vi "Actuator main.vi"() -> ()   [LabVIEW 2016]
uses:
  General/Controls/Queue modes.ctl
  General/Controls/staus modes.ctl
  General/Controls/Test settings.ctl
  General/Controls/References.ctl
  General/Controls/State control cluster.ctl
  General/Controls/States.ctl
  Actuator/Controls/Command cluster.ctl
  Actuator/Controls/Command list.ctl
  Actuator/Controls/Actuator fgv modes.ctl
  Webcam/Controls/Camera queue.ctl
  Webcam/Controls/Camera states.ctl
  DAQ/Controls/DAQ queue.ctl
  DAQ/Controls/Queue states.ctl
  <vilib>/Utility/cursorutil.llb/Set Cursor (Icon Pict).vi
  <vilib>/Platform/browser.llb/Open URL in Default Browser (string).vi
panel:
  out "Initialised":bool
  out "Trigger":bool
  in  "Load method":bool
  out "Logo 1":picture
  out "Logo 2":picture
  in  "Zero":bool
  in  "Load cell setup":bool
  in  "Abort move":bool
  in  "Initalise":bool
  in  "Snap image":bool
  in  "Test setup":bool
  in  "Camera setup":bool
  in  "Actuator setup":bool
  in  "Connect DAQ":bool
  in  "Test":bool
  in  "Connect Camera":bool
  in  "Connect Actuator":bool caption="IVIUM"
  in  "String":string=" \nLive data"
  out "LIVE DATA":dbl[](graph)
  out "LIVE DATA Force":dbl[](graph)
  in  "String 2":string=" \nActuator control"
  in  "Tab Control":enum32{"Blank", "Actuator interface"}(tab)
  in  "Limit position":dbl caption="mm" min=0.0 max=300.0 step=0.0001
  in  "Home":bool
  in  "Up":bool caption="Jog"
  in  "Down":bool
  in  "Speed":dbl=0.0001 caption="mm/s" min=0.0001 max=20.0 step=0.0001
  in  "Move absolute":bool
  in  "Target position":dbl caption="mm"
  in  "Home position":dbl caption="mm" min=0.0 max=300.0 step=0.0001
  out "Current position":dbl format="Current position - %8.4f mm"
  in  "Run method":bool
  in  "String 3":string=" \nTest data"
  out "TEST DATA":cluster{"Value":dbl, "data":dbl}(graph)
  in  "Status":string="©ReSolve Research Engineering Ltd. 2017"
  in  "Copright notice":string="Copright"
  # "Connections"
  # "Settings"
  # "Controls"
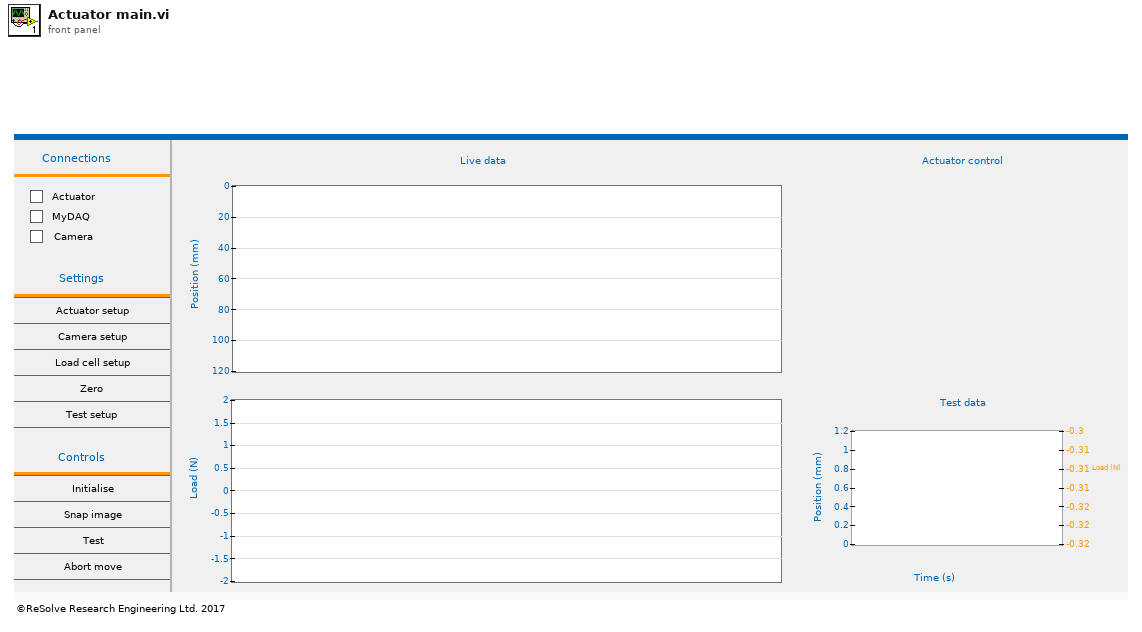
[diagram p1: front panel]
types:
  T1 = typedef "References.ctl" = cluster{"Tab Control":refnum<vi>, "Logo 1":refnum<vi>, "Logo 2":refnum<vi>, "Connect Actuator":refnum<vi>, "LIVE DATA":refnum<vi>, "Speed":refnum<vi>, "Home position":refnum<vi>, "Limit position":refnum<vi>, "Trigger":refnum<vi>, "Current position":refnum<vi>, "Connect Camera":refnum<vi>, "TEST DATA":refnum<vi>, "LIVE DATA Force":refnum<vi>, "Connect DAQ":refnum<vi>, "Initialised":refnum<vi>, "Test":refnum<vi>}
  T2 = typedef "Test settings.ctl" = cluster{"Speed (mm/s)":dbl, "Position limit":bool, "Position limit (mm)":dbl, "Load limit":bool, "Load limit (N)":dbl, "No. of repeats":u16, "Test identifier":string, "Time wait":bool, "Wait time (s)":dbl, "Trigger wait":bool, "Send trigger":bool, "Test notes":string, "Snap intervals":bool, "Time interval (s)":dbl}
  T3 = typedef "staus modes.ctl" = enum16{"Status", "Testing", "Webcam", "DAQ", "Actuator", "Initialise"}
  T4 = typedef "Queue modes.ctl" = enum16{"Initialise", "Destroy", "Get"}
  T5 = typedef "UEs.ctl" = cluster{"Read position":refnum<user-event>, "Check home":refnum<user-event>, "Record":refnum<user-event>, "Abort controller":refnum<user-event>, "Remote test":refnum<user-event>, "Test setup":refnum<user-event>, "Conditional wait":refnum<user-event>, "Abort move":refnum<user-event>, "Wait done":refnum<user-event>, "Send trigger":refnum<user-event>, "Initalising":refnum<user-event>, "Initalisation complete":refnum<user-event>}
  T6 = typedef "State control cluster.ctl" = cluster{"State":T7, "Data":variant}
  T7 = typedef "States.ctl" = enum16{"Initialise", "Actuator connection", "Get info", "Send command", "Load method", "Run method", "Save test", "Setup", "Shutdown"}
  T8 = typedef "Actuator fgv modes.ctl" = enum16{"Initalise", "COM", "Limit", "Speed", "Home", "Get"}
  T9 = typedef "Command cluster.ctl" = cluster{"Command":T10, "data":variant}
  T10 = typedef "Command list.ctl" = enum16{"", "£nabort", "getaxisno", "£getserialno", "£nidentify", "&&£setnlimit", "&£nm", "&£snv", "&£speed", "£np", "£ncal"}
  T11 = typedef "Camera queue.ctl" = cluster{"State":T12, "Data":variant}
  T12 = typedef "Camera states.ctl" = enum16{"Initialise", "Setup", "Connect", "Snap", "Close", "Shutdown"}
  T13 = typedef "DAQ queue.ctl" = cluster{"Sate":T14, "Data":variant}
  T14 = typedef "Queue states.ctl" = enum16{"Shutdown", "Save data", "Record", "Read", "Setup", "Zero", "Connect", "Initialise"}
  T15 = typedef "Default settings.ctl" = cluster{"COM port":refnum<visa-resource-name>, "Home pos":dbl, "Speed":dbl, "Limit stop":dbl}
  T16 = typedef "LVCursorListTypeDef.ctl" = cluster{"Name":string, "Color":u32, "Style":u8, "Point Style":u8, "Name Visible":bool, "Allow Drag":bool, "Cursor Mode":u32, "Plot":i32, "Index":i32, "Position":cluster{"X":dbl, "Y":dbl}, "X Scale":u32, "Y Scale":u32, "Watch Plots":i32[], "Watch All Plots":bool, "Plot Area":i32, "Label Offset":cluster{"X":dbl, "Y":dbl}}[]
  T17 = cluster{"Name":string, "Color":u32, "Style":u8, "Point Style":u8, "Name Visible":bool, "Allow Drag":bool, "Cursor Mode":u32, "Plot":i32, "Index":i32, "Position":cluster{"X":dbl, "Y":dbl}, "X Scale":u32, "Y Scale":u32, "Watch Plots":i32[], "Watch All Plots":bool, "Plot Area":i32, "Label Offset":cluster{"X":dbl, "Y":dbl}}
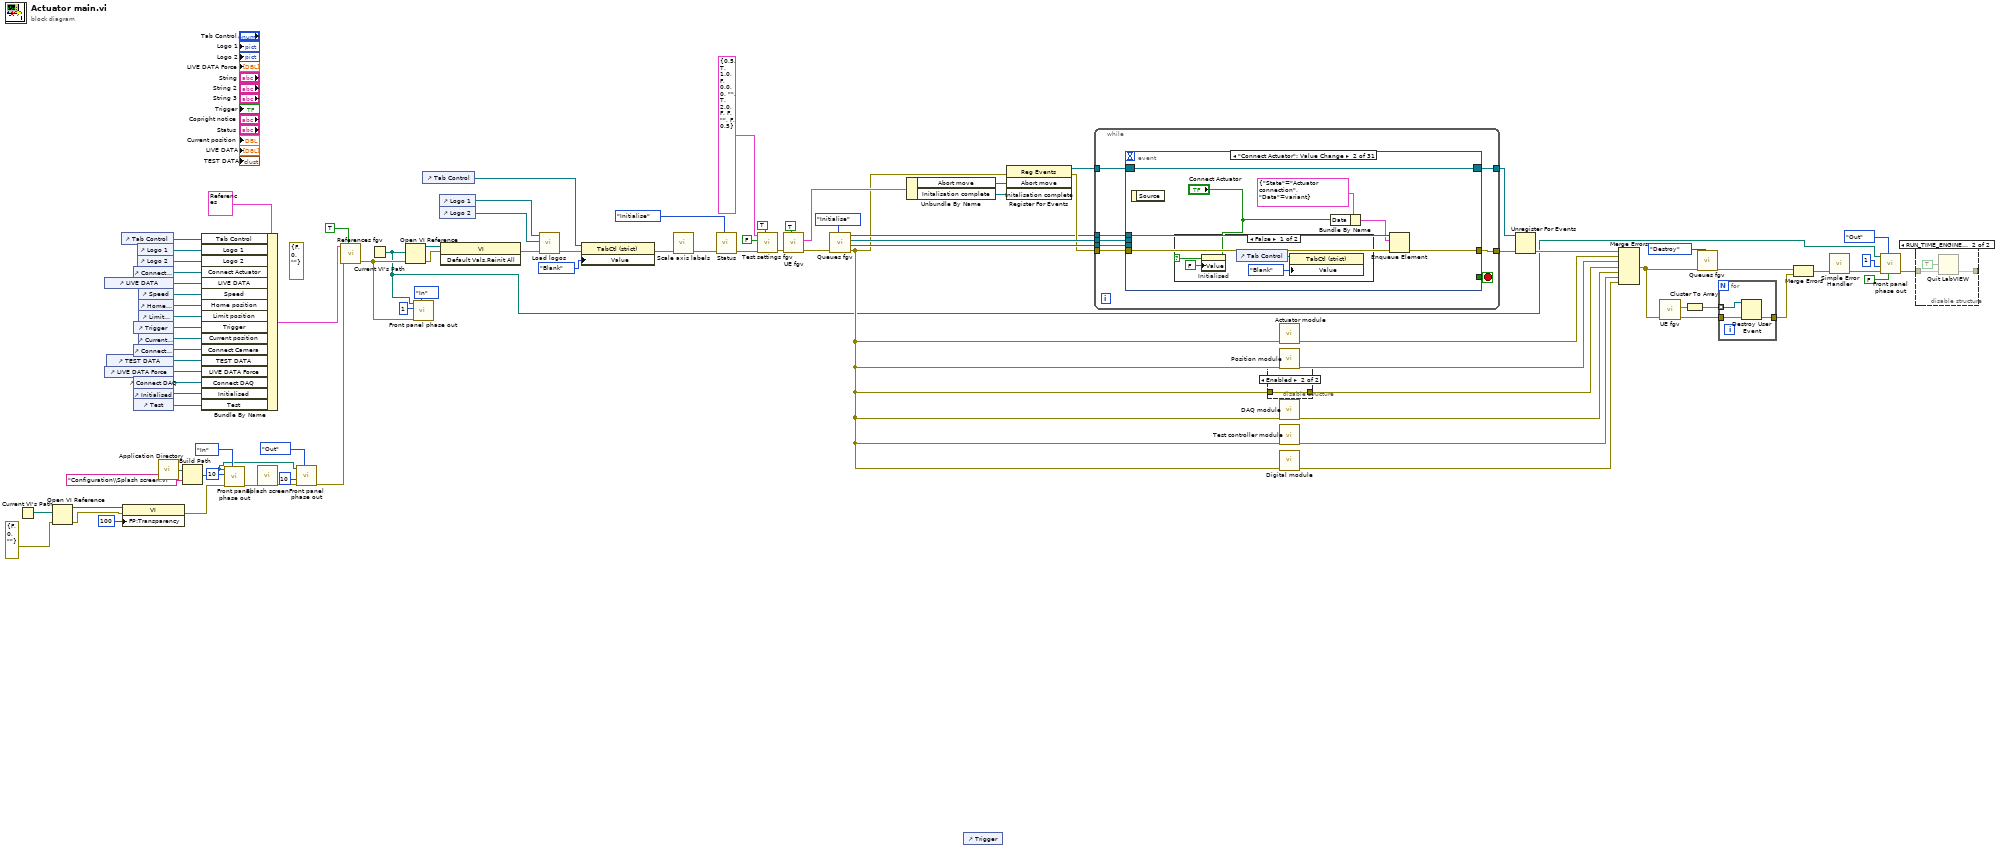
[diagram p0: block diagram]
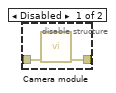
[diagram p2: hidden frame]
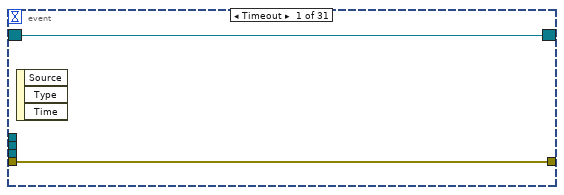
[diagram p4: hidden frame]
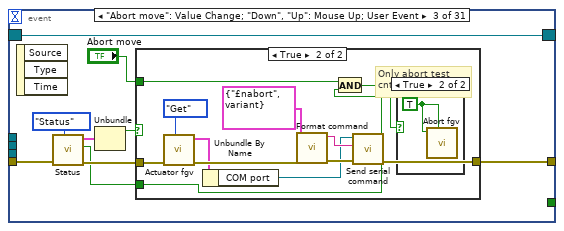
[diagram p6: hidden frame]
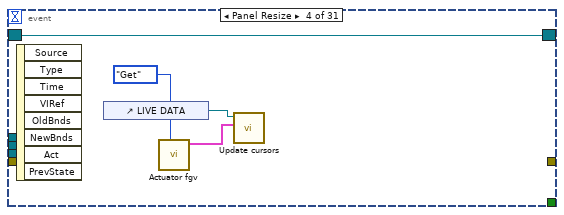
[diagram p9: hidden frame]
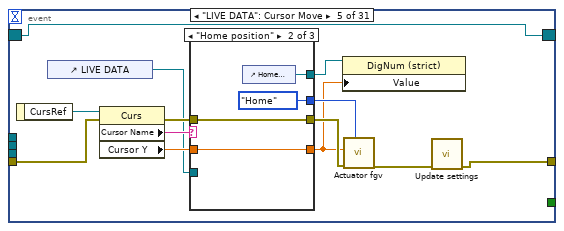
[diagram p10: hidden frame]
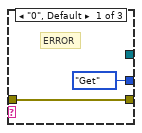
[diagram p11: hidden frame]
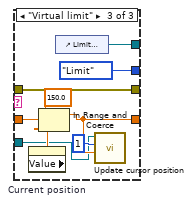
[diagram p12: hidden frame]
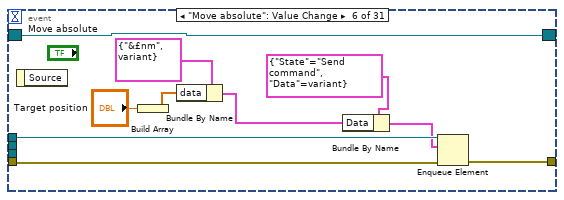
[diagram p13: hidden frame]
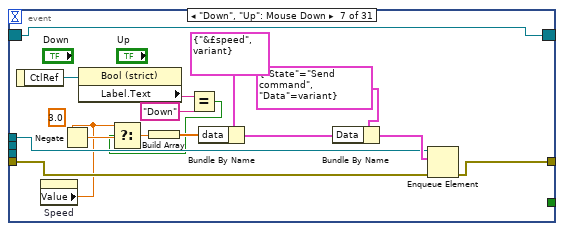
[diagram p14: hidden frame]
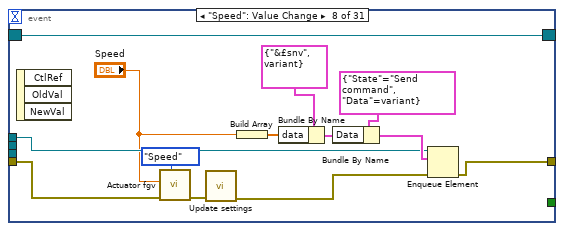
[diagram p15: hidden frame]
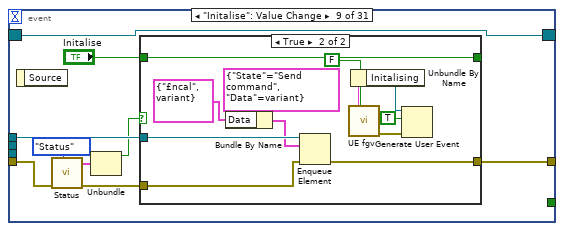
[diagram p16: hidden frame]
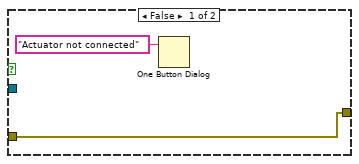
[diagram p17: hidden frame]
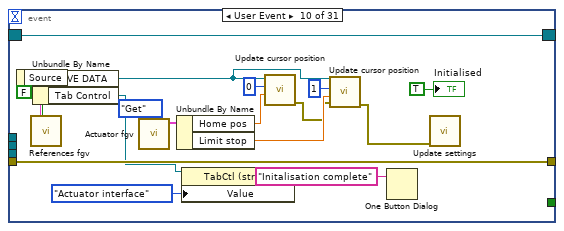
[diagram p18: hidden frame]
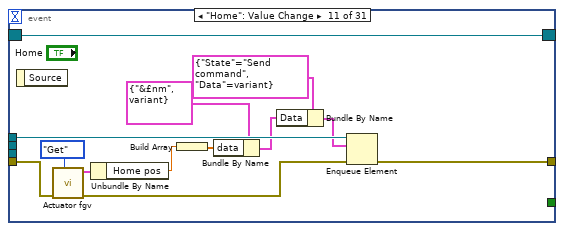
[diagram p19: hidden frame]
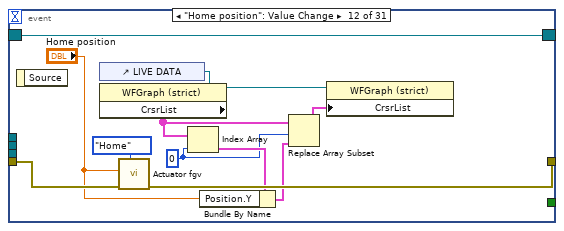
[diagram p20: hidden frame]
diagram:
  (unwired) errorcluster {"status"=FALSE, "code"=0, "source"=""} ("error in (no error)")
  n1 = Current VI's Path() -> (path=w16:path)
  n2 = Open VI Reference(vi path=w16, error in (no error)=errorcluster {"status"=FALSE, "code"=0, "source"=""}) -> (vi reference=w13:refnum<vi>, error out=w5:errorcluster)  [unwired: 4 in]
  n3 = control-ref of="LIVE DATA"() -> (w51:refnum<vi>)
  n4 = control-ref of="LIVE DATA Force"() -> (w41:refnum<vi>)
  n5 = control-ref of="TEST DATA"() -> (w42:refnum<vi>)
  n6 = control-ref of="Tab Control"() -> (w55:refnum<vi>)
  n7 = property class="VI"(reference=w13, error in=w5, "FP:Transparency"=u8 100 ("Front Panel Window:Transparency")) -> (error out=w12:errorcluster)  [unwired: 1 out]
  n8 = control-ref of="Connect Actuator"() -> (w52:refnum<vi>)
  n9 = control-ref of="Trigger"() -> (w45:refnum<vi>)
  n10 = control-ref of="Connect Camera"() -> (w43:refnum<vi>)
  n11 = control-ref of="Connect DAQ"() -> (w40:refnum<vi>)
  n12 = control-ref of="Initialised"() -> (w39:refnum<vi>)
  n13 = control-ref of="Test"() -> (w38:refnum<vi>)
  n14 = control-ref of="Logo 1"() -> (w54:refnum<vi>)
  n15 = control-ref of="Logo 2"() -> (w53:refnum<vi>)
  n16 = control-ref of="Speed"() -> (w50:refnum<vi>)
  n17 = control-ref of="Home position"() -> (w49:refnum<vi>)
  n18 = control-ref of="Limit position"() -> (w48:refnum<vi>)
  n19 = control-ref of="Current position"() -> (w44:refnum<vi>)
  n20 = call <vilib>:"Application Directory.vi"() -> ("Application Directory"=w27:path)
  n21 = Build Path(base path=w27, name or relative path="Configuration\\Splash screen.vi") -> (appended path=w22:path)
  n22 = Bundle By Name(cluster=T1 {"Tab Control"=refnum, "Logo 1"=refnum, "Logo 2"=refnum, "Connect Actuator"=refnum, "LIVE DATA"=refnum, "Speed"=refnum, "Home position"=refnum, "Limit position"=refnum, "Trigger"=refnum, "Current position"=refnum, "Connect Camera"=refnum, "TEST DATA"=refnum, "LIVE DATA Force"=refnum, "Connect DAQ"=refnum, "Initialised"=refnum, "Test"=refnum}, "Tab Control"=w55, "Logo 1"=w54, "Logo 2"=w53, "Connect Actuator"=w52, "LIVE DATA"=w51, "Speed"=w50, "Home position"=w49, "Limit position"=w48, "Trigger"=w45, "Current position"=w44, "Connect Camera"=w43, "TEST DATA"=w42, "LIVE DATA Force"=w41, "Connect DAQ"=w40, "Initialised"=w39, "Test"=w38) -> (w47:T1)
  n23 = call "Front panel phase out.vi"("Mode"=enum16{"In", "Out"}."In", "error in (no error)"=w12, "millisecond multiple In"=u32 10, "path"=w22) -> ("error out"=w24:errorcluster)  [unwired: 7 in]
  n24 = call "Splash screen.vi"("error in (no error)"=w24) -> ("error out"=w23:errorcluster)  [unwired: 10 in]
  n25 = call "Front panel phase out.vi"("Mode"=enum16{"In", "Out"}."Out", "error in (no error)"=w23, "millisecond multiple out"=u32 10, "path"=w22) -> ("error out"=w20:errorcluster)  [unwired: 7 in]
  n26 = call "References fgv.vi"("Set?"=TRUE, "error in (no error)"=w20, 11:w47) -> ("error out"=w19:errorcluster)  [unwired: 7 in, 1 out]
  n27 = Current VI's Path() -> (path=w9:path)
  n28 = Open VI Reference(vi path=w9, error in (no error)=w19) -> (vi reference=w18:refnum<vi>, error out=w89:errorcluster)  [unwired: 4 in]
  n29 = call "Front panel phase out.vi"("Mode"=enum16{"In", "Out"}."In", "error in (no error)"=w19, "millisecond multiple In"=u32 1, "path"=w9) -> ()  [unwired: 7 in, 1 out]
  n30 = control-ref of="Tab Control"() -> (w83:refnum<vi>)
  n31 = control-ref of="Logo 1"() -> (w65:refnum<vi>)
  n32 = control-ref of="Logo 2"() -> (w64:refnum<vi>)
  n33 = invoke class="VI" method="Default Vals.Reinit All"(reference=w18, error in=w89) -> (error out=w33:errorcluster)  [unwired: 1 in, 2 out]
  n34 = call "Load logos.vi"("error in (no error)"=w33, "Logo 2"=w64, "Logo 1"=w65) -> ("error out"=w63:errorcluster)  [unwired: 6 in, 2 out]
  n35 = property class="TabCtl (strict)"(reference=w83, error in=w63, "Value"=enum32{"Blank", "Actuator interface"}."Blank") -> (error out=w32:errorcluster)  [unwired: 1 out]
  n36 = call "Scale axis labels.vi"("error in (no error)"=w32) -> ("error out"=w31:errorcluster)  [unwired: 10 in]
  n37 = call "Status.vi"("Mode"=staus_modes."Initialise", "error in (no error)"=w31) -> ("error out"=w70:errorcluster)  [unwired: 7 in, 2 out]
  n38 = call "Test settings fgv.vi"("Set?"=TRUE, "error in (no error)"=w70, "Settings selected?"=FALSE, "Test settings"=T2 {"Speed (mm/s)"=0.5, "Position limit"=TRUE, "Position limit (mm)"=1.0, "Load limit"=FALSE, "Load limit (N)"=0.0, "No. of repeats"=0, "Test identifier"="", "Time wait"=TRUE, "Wait time (s)"=2.0, "Trigger wait"=FALSE, "Send trigger"=FALSE, "Test notes"="", "Snap intervals"=FALSE, "Time interval (s)"=0.5}) -> ("error out"=w37:errorcluster)  [unwired: 5 in, 2 out]
  n39 = call "UE fgv.vi"("Set?"=TRUE, "error in (no error)"=w37) -> ("error out"=w36:errorcluster, "UEs"=w35:T5)  [unwired: 7 in, 1 out]
  n40 = call "Queues fgv.vi"("Modes"=Queue_modes."Initialise", "error in (no error)"=w36) -> ("error in (no error) 2"=w34:errorcluster, "DAQ"=w81:refnum<queue>, "Camera"=w87:refnum<queue>, "Ivium"=w61:refnum<queue>)  [unwired: 6 in]
  n41 = Unbundle By Name(w35) -> ("Abort move"=w72:refnum<user-event>, "Initalisation complete"=w1:refnum<user-event>)
  n42 = control-ref of="Trigger"() -> ()  [unwired: 1 out]
  n43 = register-events(error in=w34, w72, w1) -> (reference out=w71:refnum<event-registration>, error out=w66:errorcluster)  [unwired: 1 in]
  n44 = while {
    tunnel: w66 -> [w96]
    tunnel: [w95] -> w59
    tunnel: w61 -> [w94]
    tunnel: w87 -> [w93]
    tunnel: w81 -> [w92]
    tunnel: w71 -> [w91]
    tunnel: [w90] -> w57
    stop <- w97 stop-if-true
    n45 = event shown="[1] \"Connect Actuator\": Value Change" {
      selector: w91 -> [w98 w101 w111 w133 w137 w165 w175 w191 w204 w243 w244 w257 w269 w282 w287 w292 w299 w306 w311 w316 w321 w326 w331 w339 w347 w351 w355 w359 w363 w368 w373]
      dyn-events: [w98 w101 w111 w133 w137 w165 w175 w191 w204 w243 w244 w257 w269 w282 w287 w292 w299 w306 w311 w316 w321 w326 w331 w339 w347 w351 w355 w359 w363 w368 w373] -> w90
      timeout: _ -> [_ _ _ _ _ _ _ _ _ _ _ _ _ _ _ _ _ _ _ _ _ _ _ _ _ _ _ _ _ _ _]
      tunnel: [_ _ _ _ _ _ _ _ _ _ _ _ _ _ _ _ _ _ _ _ _ _ _ _ _ _ _ _ _ _ TRUE] -> w97
      tunnel: w96 -> [w99 w106 w115 _ w143 w166 w184 w196 w210 w242 w249 w268 w281 w283 w291 w298 w305 w310 w315 w320 w325 w330 w335 w343 w349 w353 w356 w362 w366 w371 w377]
      tunnel: [w99 w104 w118 _ w141 w171 w185 w198 w212 w242 w256 w266 w277 w285 w289 w297 w304 w309 w314 w319 w324 w327 w338 w346 w348 w352 w357 w361 w365 w370 w380] -> w95
      tunnel: w94 -> [_ w105 _ _ _ w170 w183 w197 w211 _ w255 _ _ w286 w290 _ _ _ _ _ _ w329 _ _ _ _ _ _ _ _ w390]
      tunnel: w93 -> [_ _ _ _ _ _ _ _ _ _ _ _ _ _ _ w295 _ w308 _ _ w323 _ _ _ _ _ _ _ _ _ w388]
      tunnel: w92 -> [_ _ _ _ _ _ _ _ _ _ _ _ _ _ _ _ w301 _ w313 w318 _ _ _ _ _ _ _ _ _ _ w386]
      event Timeout {
        n46 = event-data() -> ()  [unwired: 1 in, 3 out]
      }
      event "Connect Actuator": Value Change {
        n47 = event-data() -> ()  [unwired: 1 in, 1 out]
        n48 = case shown="False" "Connect Actuator" {
          frame False {
            n49 = property on="Initialised" class="Bool (strict)"("Value"=FALSE ("Initialised")) -> ()  [unwired: 2 in, 2 out]
            n50 = control-ref of="Tab Control"() -> (w109:refnum<vi>)
            n51 = property class="TabCtl (strict)"(reference=w109, "Value"=enum32{"Blank", "Actuator interface"}."Blank") -> ()  [unwired: 1 in, 2 out]
          }
          frame True {
          }
        }
        n52 = Bundle By Name(cluster=T6 {"State"=enum."Actuator connection", "Data"=variant} ("State control"), "Data"="Connect Actuator") -> (w102:T6)
        n53 = Enqueue Element(queue=w105, element=w102, error in (no error)=w106) -> (error out=w104:errorcluster)  [unwired: 1 in, 2 out]
      }
      event "Abort move": Value Change; "Down", "Up": Mouse Up; User Event {
        n54 = event-data() -> ()  [unwired: 1 in, 3 out]
        n55 = call "Status.vi"("Mode"=staus_modes."Status", "error in (no error)"=w115) -> ("error out"=w114:errorcluster, "Testing"=w112:bool, "Connections"=w116:cluster{"Data":bool, "Data":bool, "Data":bool})  [unwired: 7 in]
        n56 = Unbundle(w116) -> ("Data"=w113:bool)  [unwired: 2 out]
        n57 = case shown="True" w113 {
          tunnel: [w119 w129] -> w118
          tunnel: w114 -> [w119 w128]
          tunnel: w112 -> [_ w121]
          tunnel: "Abort move" -> [_ w122]
          frame False {
          }
          frame True {
            # "Only abort test \ncntrl from button"
            n58 = call "Actuator fgv.vi"("Enum"=Actuator_fgv_modes."Get", "error in (no error)"=w128) -> ("error out"=w127:errorcluster, "Cluster out"=w125:T15)  [unwired: 8 in]
            n59 = Unbundle By Name(w125) -> ("COM port"=w123:refnum<visa-resource-name>)
            n60 = call "Format command.vi"("error in (no error)"=w127, "Cluster"=T9 {"Command"=enum."£nabort", "data"=variant}) -> ("error out"=w131:errorcluster, "String"=w130:string)  [unwired: 8 in]
            n61 = And(x=w122, y=w121) -> (x .and. y?=w120:bool)
            n62 = call "Send serial command.vi"("error IO"=w131, "Send string"=w130, "VISA resource name out"=w123) -> ("error out"=w129:errorcluster)  [unwired: 6 in, 2 out]
            n63 = case shown="True" w120 {
              frame False {
              }
              frame True {
                w132 = TRUE ("Set?")
                n64 = call "Abort fgv.vi"("Set?"=w132, "Value"=w132) -> ()  [unwired: 9 in, 1 out]
              }
            }
          }
        }
      }
      event Panel Resize {
        n65 = event-data() -> ()  [unwired: 1 in, 8 out]
        n66 = control-ref of="LIVE DATA"() -> (w134:refnum<vi>)
        n67 = call "Actuator fgv.vi"("Enum"=Actuator_fgv_modes."Get") -> ("Cluster out"=w135:T15)  [unwired: 9 in, 1 out]
        n68 = call "Update cursors.vi"("Cluster in"=w135, "LIVE DATA 3"=w134) -> ()  [unwired: 9 in, 1 out]
      }
      event "LIVE DATA": Cursor Move {
        n69 = event-data() -> ("CursRef"=w149:refnum<vi>)  [unwired: 1 in]
        n70 = control-ref of="LIVE DATA"() -> (w138:refnum<vi>)
        n71 = property class="Curs"(reference=w149, error in=w143) -> (error out=w145:errorcluster, "Cursor Name"=w148:string, "Cursor Y"=w147:dbl)  [unwired: 1 out]
        n72 = case shown="\"Home position\"" w148 {
          tunnel: w147 -> [_ w155 w161]
          tunnel: [_ w155 w158] -> w139
          tunnel: [Actuator_fgv_modes."Get" ("Enum") Actuator_fgv_modes."Home" ("Enum") Actuator_fgv_modes."Limit" ("Enum")] -> w146
          tunnel: w145 -> [w150 w153 w163]
          tunnel: [w150 w153 w163] -> w144
          tunnel: [_ w152 w162] -> w140
          tunnel: w138 -> [_ _ w156]
          frame "0", Default {
            # "ERROR"
          }
          frame "Home position" {
            n73 = control-ref of="Home position"() -> (w152:refnum<vi>)
          }
          frame "Virtual limit" {
            n74 = property on="Current position" class="DigNum (strict)"() -> ("Value"=w160:dbl)  [unwired: 2 in, 2 out]
            n75 = In Range and Coerce(upper limit=150.0, x=w161, lower limit=w160) -> (coerced(x)=w158:dbl)  [unwired: 1 out]
            n76 = control-ref of="Limit position"() -> (w162:refnum<vi>)
            n77 = call "Update cursor position.vi"("Position Y"=w158, "index"=1, "LIVE DATA 3"=w156) -> ()  [unwired: 8 in, 1 out]
          }
        }
        n78 = property class="DigNum (strict)"(reference=w140, "Value"=w139) -> ()  [unwired: 1 in, 2 out]
        n79 = call "Actuator fgv.vi"("Enum"=w146, "error in (no error)"=w144, "Data"=w139) -> ("error out"=w142:errorcluster)  [unwired: 7 in, 1 out]
        n80 = call "Update settings.vi"("error in (no error)"=w142) -> ("error out"=w141:errorcluster)  [unwired: 10 in]
      }
      event "Move absolute": Value Change {
        n81 = event-data() -> ()  [unwired: 1 in, 1 out]
        n82 = Build Array("Target position") -> (w172:dbl[])
        n83 = Bundle By Name(cluster=T9 {"Command"=enum."&£nm", "data"=variant} ("Cluster"), "data"=w172) -> (w168:T9)
        n84 = Bundle By Name(cluster=T6 {"State"=enum."Send command", "Data"=variant} ("element"), "Data"=w168) -> (w167:T6)
        n85 = Enqueue Element(queue=w170, element=w167, error in (no error)=w166) -> (error out=w171:errorcluster)  [unwired: 1 in, 2 out]
      }
      event "Down", "Up": Mouse Down {
        (unwired) 3.0
        n86 = event-data() -> ("CtlRef"=w180:refnum<vi>)  [unwired: 1 in]
        n87 = property on="Speed" class="DigNum (strict)"() -> ("Value"=w176:dbl)  [unwired: 2 in, 2 out]
        n88 = Negate(x=w176) -> (-x=w182:dbl)
        n89 = property class="Bool (strict)"(reference=w180) -> ("Label.Text"=w179:string)  [unwired: 1 in, 2 out]
        n90 = Equal?(x=w179, y="Down") -> (x = y?=w177:bool)
        n91 = Select(t=w176, s=w177, f=w182) -> (s? t:f=w181:dbl)
        n92 = Build Array(w181) -> (w190:dbl[])
        n93 = Bundle By Name(cluster=T9 {"Command"=enum."&£speed", "data"=variant} ("Cluster"), "data"=w190) -> (w186:T9)
        n94 = Bundle By Name(cluster=T6 {"State"=enum."Send command", "Data"=variant} ("element"), "Data"=w186) -> (w187:T6)
        n95 = Enqueue Element(queue=w183, element=w187, error in (no error)=w184) -> (error out=w185:errorcluster)  [unwired: 1 in, 2 out]
      }
      event "Speed": Value Change {
        n96 = event-data() -> ()  [unwired: 1 in, 3 out]
        n97 = call "Actuator fgv.vi"("Enum"=Actuator_fgv_modes."Speed", "error in (no error)"=w196, "Data"="Speed") -> ("error out"=w195:errorcluster)  [unwired: 7 in, 1 out]
        n98 = call "Update settings.vi"("error in (no error)"=w195) -> ("error out"=w194:errorcluster)  [unwired: 10 in]
        n99 = Build Array("Speed") -> (w203:dbl[])
        n100 = Bundle By Name(cluster=T9 {"Command"=enum."&£snv", "data"=variant} ("Cluster"), "data"=w203) -> (w199:T9)
        n101 = Bundle By Name(cluster=T6 {"State"=enum."Send command", "Data"=variant} ("element"), "Data"=w199) -> (w200:T6)
        n102 = Enqueue Element(queue=w197, element=w200, error in (no error)=w194) -> (error out=w198:errorcluster)  [unwired: 1 in, 2 out]
      }
      event "Initalise": Value Change {
        n103 = event-data() -> ()  [unwired: 1 in, 1 out]
        n104 = call "Status.vi"("Mode"=staus_modes."Status", "error in (no error)"=w210) -> ("error out"=w209:errorcluster, "Connections"=w208:cluster{"Data":bool, "Data":bool, "Data":bool})  [unwired: 7 in, 1 out]
        n105 = Unbundle(w208) -> ("Data"=w206:bool)  [unwired: 2 out]
        n106 = case shown="True" w206 {
          tunnel: [w213 w215] -> w212
          tunnel: w211 -> [_ w226]
          tunnel: w209 -> [w213 w222]
          tunnel: "Initalise" -> [_ w221]
          tunnel: [_ w221] -> _
          frame False {
            n107 = One Button Dialog(message="Actuator not connected") -> ()  [unwired: 1 in, 1 out]
          }
          frame True {
            n108 = Bundle By Name(cluster=T6 {"State"=enum."Send command", "Data"=variant} ("element"), "Data"=T9 {"Command"=enum."£ncal", "data"=variant} ("Cluster")) -> (w223:T6)
            n109 = Enqueue Element(queue=w226, element=w223, error in (no error)=w222) -> (error out=w215:errorcluster)  [unwired: 1 in, 2 out]
            n110 = call "UE fgv.vi"("Set?"=FALSE) -> ("error out"=w218:errorcluster, "UEs"=w219:T5)  [unwired: 8 in, 1 out]
            n111 = Unbundle By Name(w219) -> ("Initalising"=w217:refnum<user-event>)
            n112 = Generate User Event(user event=w217, event data cluster=TRUE ("event data"), error in=w218) -> ()  [unwired: 1 in, 2 out]
          }
        }
      }
      event User Event {
        n113 = event-data() -> ()  [unwired: 1 in, 1 out]
        n114 = call "References fgv.vi"("Set?"=FALSE) -> ("Cluster"=w239:T1)  [unwired: 9 in, 1 out]
        n115 = Unbundle By Name(w239) -> ("LIVE DATA"=w233:refnum<vi>, "Tab Control"=w238:refnum<vi>)
        n116 = call "Actuator fgv.vi"("Enum"=Actuator_fgv_modes."Get") -> ("Cluster out"=w235:T15)  [unwired: 9 in, 1 out]
        n117 = Unbundle By Name(w235) -> ("Home pos"=w234:dbl, "Limit stop"=w231:dbl)
        n118 = property class="TabCtl (strict)"(reference=w238, "Value"=enum32{"Blank", "Actuator interface"}."Actuator interface") -> ()  [unwired: 1 in, 2 out]
        n119 = call "Update cursor position.vi"("Position Y"=w234, "index"=0, "LIVE DATA 3"=w233) -> ("error out"=w229:errorcluster)  [unwired: 8 in]
        n120 = call "Update cursor position.vi"("error in (no error)"=w229, "Position Y"=w231, "index"=1, "LIVE DATA 3"=w233) -> ("error out"=w230:errorcluster)  [unwired: 7 in]
        n121 = One Button Dialog(message="Initalisation complete") -> ()  [unwired: 1 in, 1 out]
        n122 = call "Update settings.vi"("error in (no error)"=w230) -> ()  [unwired: 10 in, 1 out]
        "Initialised" <- TRUE ("Initialised")
      }
      event "Home": Value Change {
        n123 = event-data() -> ()  [unwired: 1 in, 1 out]
        n124 = call "Actuator fgv.vi"("Enum"=Actuator_fgv_modes."Get", "error in (no error)"=w249) -> ("error out"=w248:errorcluster, "Cluster out"=w246:T15)  [unwired: 8 in]
        n125 = Unbundle By Name(w246) -> ("Home pos"=w245:dbl)
        n126 = Build Array(w245) -> (w250:dbl[])
        n127 = Bundle By Name(cluster=T9 {"Command"=enum."&£nm", "data"=variant} ("Cluster"), "data"=w250) -> (w251:T9)
        n128 = Bundle By Name(cluster=T6 {"State"=enum."Send command", "Data"=variant} ("element"), "Data"=w251) -> (w253:T6)
        n129 = Enqueue Element(queue=w255, element=w253, error in (no error)=w248) -> (error out=w256:errorcluster)  [unwired: 1 in, 2 out]
      }
      event "Home position": Value Change {
        w262 = 0 ("index")
        n130 = event-data() -> ()  [unwired: 1 in, 1 out]
        n131 = control-ref of="LIVE DATA"() -> (w265:refnum<vi>)
        n132 = property class="WFGraph (strict)"(reference=w265) -> (reference out=w260:refnum<vi>, "CrsrList"=w263:T16)  [unwired: 1 in, 1 out]
        n133 = call "Actuator fgv.vi"("Enum"=Actuator_fgv_modes."Home", "error in (no error)"=w268, "Data"="Home position") -> ("error out"=w266:errorcluster)  [unwired: 7 in, 1 out]
        n134 = Index Array(array=w263, index=w262) -> (element=w264:T17)
        n135 = Bundle By Name(cluster=w264, "Position.Y"="Home position") -> (w261:T17)
        n136 = Replace Array Subset(array=w263, new element=w261, index=w262) -> (w259:T16)
        n137 = property class="WFGraph (strict)"(reference=w260, "CrsrList"=w259) -> ()  [unwired: 1 in, 2 out]
      }
      event "Limit position": Value Change {
        n138 = event-data() -> ()  [unwired: 1 in, 1 out]
        n139 = property on="Current position" class="DigNum (strict)"() -> ("Value"=w275:dbl)  [unwired: 2 in, 2 out]
        n140 = In Range and Coerce(upper limit=150.0, x="Limit position", lower limit=w275) -> (coerced(x)=w272:dbl)  [unwired: 1 out]
        n141 = control-ref of="LIVE DATA"() -> (w279:refnum<vi>)
        n142 = call "Actuator fgv.vi"("Enum"=Actuator_fgv_modes."Limit", "error in (no error)"=w281, "Data"=w272) -> ("error out"=w271:errorcluster)  [unwired: 7 in, 1 out]
        n143 = call "Update cursor position.vi"("error in (no error)"=w271, "Position Y"=w272, "index"=1, "LIVE DATA 3"=w279) -> ("error out"=w270:errorcluster)  [unwired: 7 in]
        n144 = property on="Limit position" class="DigNum (strict)"(error in=w270, "Value"=w272) -> (error out=w273:errorcluster)  [unwired: 1 in, 1 out]
        n145 = call "Update settings.vi"("error in (no error)"=w273) -> ("error out"=w277:errorcluster)  [unwired: 10 in]
      }
      event "Load method": Value Change {
        n146 = event-data() -> ()  [unwired: 1 in, 1 out]
        n147 = Enqueue Element(queue=w286, element=T6 {"State"=enum."Load method", "Data"=variant} ("State control"), error in (no error)=w283) -> (error out=w285:errorcluster)  [unwired: 1 in, 2 out]
      }
      event "Run method": Value Change {
        n148 = event-data() -> ()  [unwired: 1 in, 1 out]
        n149 = Enqueue Element(queue=w290, element=T6 {"State"=enum."Run method", "Data"=variant} ("State control"), error in (no error)=w291) -> (error out=w289:errorcluster)  [unwired: 1 in, 2 out]
      }
      event "Connect Camera": Value Change {
        n150 = event-data() -> ()  [unwired: 1 in, 1 out]
        n151 = Bundle By Name(cluster=T11 {"State"=enum."Connect", "Data"=variant}, "Data"="Connect Camera") -> (w296:T11)
        n152 = Enqueue Element(queue=w295, element=w296, error in (no error)=w298) -> (error out=w297:errorcluster)  [unwired: 1 in, 2 out]
      }
      event "Connect DAQ": Value Change {
        n153 = event-data() -> ()  [unwired: 1 in, 1 out]
        n154 = Bundle By Name(cluster=T13 {"Sate"=enum."Connect", "Data"=variant} ("DAQ Queue"), "Data"="Connect DAQ") -> (w303:T13)
        n155 = Enqueue Element(queue=w301, element=w303, error in (no error)=w305) -> (error out=w304:errorcluster)  [unwired: 1 in, 2 out]
      }
      event "Camera setup": Value Change {
        n156 = event-data() -> ()  [unwired: 1 in, 6 out]
        n157 = Enqueue Element(queue=w308, element=T11 {"State"=enum."Setup", "Data"=variant}, error in (no error)=w310) -> (error out=w309:errorcluster)  [unwired: 1 in, 2 out]
      }
      event "Load cell setup": Value Change {
        n158 = event-data() -> ()  [unwired: 1 in, 1 out]
        n159 = Enqueue Element(queue=w313, element=T13 {"Sate"=enum."Setup", "Data"=variant}, error in (no error)=w315) -> (error out=w314:errorcluster)  [unwired: 1 in, 2 out]
      }
      event "Zero": Value Change {
        n160 = event-data() -> ()  [unwired: 1 in, 1 out]
        n161 = Enqueue Element(queue=w318, element=T13 {"Sate"=enum."Zero", "Data"=variant}, error in (no error)=w320) -> (error out=w319:errorcluster)  [unwired: 1 in, 2 out]
      }
      event "Snap image": Value Change {
        n162 = event-data() -> ()  [unwired: 1 in, 1 out]
        n163 = Enqueue Element(queue=w323, element=T11 {"State"=enum."Snap", "Data"=variant}, error in (no error)=w325) -> (error out=w324:errorcluster)  [unwired: 1 in, 2 out]
      }
      event "Actuator setup": Value Change {
        n164 = event-data() -> ()  [unwired: 1 in, 1 out]
        n165 = Enqueue Element(queue=w329, element=T6 {"State"=enum."Setup", "Data"=variant} ("State control"), error in (no error)=w330) -> (error out=w327:errorcluster)  [unwired: 1 in, 2 out]
      }
      event "Test setup": Value Change {
        n166 = event-data() -> ()  [unwired: 1 in, 1 out]
        n167 = call "UE fgv.vi"("Set?"=FALSE, "error in (no error)"=w335) -> ("error out"=w334:errorcluster, "UEs"=w336:T5)  [unwired: 7 in, 1 out]
        n168 = Unbundle By Name(w336) -> ("Test setup"=w332:refnum<user-event>)
        n169 = Generate User Event(user event=w332, event data cluster=TRUE ("event data"), error in=w334) -> (error out=w338:errorcluster)  [unwired: 1 in, 1 out]
      }
      event "Test": Value Change {
        n170 = event-data() -> ()  [unwired: 1 in, 1 out]
        n171 = call "UE fgv.vi"("Set?"=FALSE, "error in (no error)"=w343) -> ("error out"=w342:errorcluster, "UEs"=w344:T5)  [unwired: 7 in, 1 out]
        n172 = Unbundle By Name(w344) -> ("Remote test"=w340:refnum<user-event>)
        n173 = Generate User Event(user event=w340, event data cluster=TRUE ("event data"), error in=w342) -> (error out=w346:errorcluster)  [unwired: 1 in, 1 out]
      }
      event "Logo 1", "Logo 2": Mouse Enter {
        n174 = event-data() -> ()  [unwired: 1 in, 4 out]
        n175 = call-poly <vilib>:"Set Cursor.vi"("error in (no error)"=w349, "icon"=u16 6) -> ("error out"=w348:errorcluster)  [unwired: 8 in, 1 out]
      }
      event "Logo 1", "Logo 2": Mouse Leave {
        n176 = event-data() -> ()  [unwired: 1 in, 4 out]
        n177 = call-poly <vilib>:"Set Cursor.vi"("error in (no error)"=w353, "icon"=u16 0) -> ("error out"=w352:errorcluster)  [unwired: 8 in, 1 out]
      }
      event "Logo 1": Mouse Up {
        n178 = event-data() -> ()  [unwired: 1 in, 1 out]
        n179 = call-poly <vilib>:"Open URL in Default Browser.vi"("error in (no error)"=w356, "URL"="http://www.resolve-re.co.uk/") -> ("error out"=w357:errorcluster)  [unwired: 4 in, 1 out]
      }
      event "Logo 2": Mouse Up {
        n180 = event-data() -> ()  [unwired: 1 in, 1 out]
        n181 = call-poly <vilib>:"Open URL in Default Browser.vi"("error in (no error)"=w362, "URL"="https://www.engineering.leeds.ac.uk/functional-surfaces/") -> ("error out"=w361:errorcluster)  [unwired: 4 in, 1 out]
      }
      event "Actuator setup", "Camera setup", "Test setup", "Snap image", "Test", "Move absolute", "Home", "Initalise", "Abort move", "Load cell setup", "Zero": Mouse Enter {
        (unwired) cluster{u32, u32}[] [{9868950, 16765843}, {0, 0}, {4934475, 8350025}, {8355711, 8355711}] ("Colors [4]")
        (unwired) cluster{u32, u32}[] [{9868950, 16750592}, {0, 0}, {4934475, 8342528}, {8355711, 8355711}] ("Colors [4]")
        n182 = event-data() -> ("CtlRef"=w367:refnum<vi>)  [unwired: 1 in, 3 out]
        n183 = property class="Bool"(reference=w367, error in=w366, "Colors [4]"=cluster{u32, u32}[] [{11776947, 16765843}, {11776947, 16750592}, {5855577, 8350025}, {5855577, 8342528}]) -> (error out=w365:errorcluster)  [unwired: 1 out]
      }
      event "Actuator setup", "Camera setup", "Test setup", "Snap image", "Test", "Move absolute", "Home", "Initalise", "Abort move", "Load cell setup", "Zero": Mouse Leave {
        (unwired) cluster{u32, u32}[] [{9868950, 16777216}, {0, 0}, {4934475, 16777216}, {8355711, 8355711}] ("Colors [4]")
        n184 = event-data() -> ("CtlRef"=w372:refnum<vi>)  [unwired: 1 in, 3 out]
        n185 = property class="Bool"(reference=w372, error in=w371, "Colors [4]"=cluster{u32, u32}[] [{9868950, 16777216}, {11776947, 16750592}, {4934475, 16777216}, {5855577, 8342528}]) -> (error out=w370:errorcluster)  [unwired: 1 out]
      }
      event Panel Close? {
        n186 = event-data() -> ()  [unwired: 1 in, 1 out]
        n187 = call "UE fgv.vi"("Set?"=FALSE, "error in (no error)"=w377) -> ("error out"=w376:errorcluster, "UEs"=w379:T5)  [unwired: 7 in, 1 out]
        n188 = Unbundle By Name(w379) -> ("Abort controller"=w375:refnum<user-event>)
        n189 = Generate User Event(user event=w375, event data cluster=TRUE ("Discard?"), error in=w376) -> (error out=w382:errorcluster)  [unwired: 1 in, 1 out]
        n190 = Enqueue Element(queue=w386, element=T13 {"Sate"=enum."Shutdown", "Data"=variant}, error in (no error)=w382) -> (error out=w385:errorcluster)  [unwired: 1 in, 2 out]
        n191 = Enqueue Element(queue=w388, element=T11 {"State"=enum."Shutdown", "Data"=variant}, error in (no error)=w385) -> (error out=w381:errorcluster)  [unwired: 1 in, 2 out]
        n192 = Enqueue Element(queue=w390, element=T6 {"State"=enum."Shutdown", "Data"=variant}, error in (no error)=w381) -> (error out=w380:errorcluster)  [unwired: 1 in, 2 out]
        n193 = event-data("Discard?"=TRUE) -> ()  [unwired: 1 in, 1 out]
      }
    }
  }
  n194 = disable-structure shown="Enabled" {
    disable-tunnel: [w393 w394] -> w78
    disable-tunnel: w34 -> [w392 w394]
    frame Disabled {
      n195 = call "Camera module.vi"("error in (no error)"=w392) -> ("error out"=w393:errorcluster)  [unwired: 10 in]
    }
    frame Enabled {
    }
  }
  n196 = call "Actuator module.vi"("error in (no error)"=w34) -> ("error out"=w80:errorcluster)  [unwired: 10 in]
  n197 = call "Position module.vi"("error in (no error)"=w34) -> ("error out"=w60:errorcluster)  [unwired: 10 in]
  n198 = call "DAQ module.vi"("error in (no error)"=w34) -> ("error out"=w85:errorcluster)  [unwired: 10 in]
  n199 = call "Test controller module.vi"("error in (no error)"=w34) -> ("error out"=w62:errorcluster)  [unwired: 10 in]
  n200 = call "Digital module.vi"("error in (no error)"=w34) -> ("error out"=w77:errorcluster)  [unwired: 10 in]
  n201 = Unregister For Events(event registration refnum=w57, error in=w59) -> (error out=w58:errorcluster)
  n202 = Merge Errors(w58, w80, w60, w78, w85, w62, w77) -> (w76:errorcluster)
  n203 = call "UE fgv.vi"("error in (no error)"=w76) -> ("error out"=w73:errorcluster, "UEs"=w75:T5)  [unwired: 8 in, 1 out]
  n204 = Cluster To Array(cluster=w75) -> (array=w74:refnum<user-event>[])
  n205 = call "Queues fgv.vi"("Modes"=Queue_modes."Destroy", "error in (no error)"=w76) -> ("error in (no error) 2"=w30:errorcluster)  [unwired: 6 in, 3 out]
  n206 = for {
    tunnel: w74 -> [w397] mode=indexing
    tunnel: w73 -> [w396]
    tunnel: [w395] -> w29
    n207 = Destroy User Event(user event=w397, error in=w396) -> (error out=w395:errorcluster)
  }
  n208 = Merge Errors(w30, w29) -> (w28:errorcluster)
  n209 = call <vilib>:"Simple Error Handler.vi"("error in (no error)"=w28) -> ("error out"=w17:errorcluster)  [unwired: 4 in, 4 out]
  n210 = call "Front panel phase out.vi"("close?"=FALSE, "Mode"=enum16{"In", "Out"}."Out", "error in (no error)"=w17, "millisecond multiple out"=u32 1, "path"=w9) -> ("error out"=w10:errorcluster)  [unwired: 6 in]
  n211 = disable-structure shown="RUN_TIME_ENGINE==True" {
    disable-tunnel: w10 -> [w398 w399]
    disable-tunnel: [w398 w399] -> _
    frame condition #0 (active) {
    }
    frame condition #1 {
      n212 = Quit LabVIEW(quit? (T)=TRUE) -> ()
    }
  }
